vi "Find Supporting.vi"(11 "Bricks in":T1(array[cluster])) -> (3 "Bricks out":T1(array[cluster]))   [LabVIEW 2023, in "d22.lvlib"]
uses:
  d22.lvlib
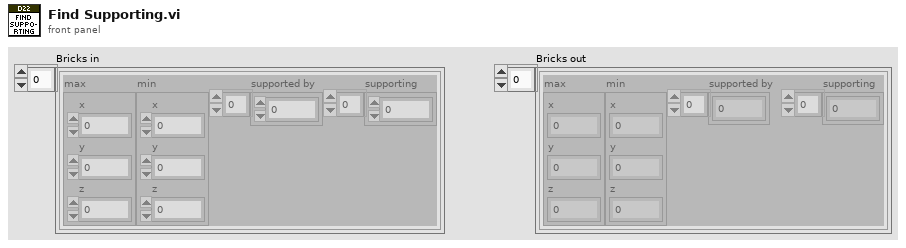
[diagram p1: front panel]
types:
  T1 = cluster{"max":cluster{"x":i32, "y":i32, "z":i32}, "min":cluster{"x":i32, "y":i32, "z":i32}, "supported by":i32[], "supporting":i32[]}[]
  T2 = cluster{"max":cluster{"x":i32, "y":i32, "z":i32}, "min":cluster{"x":i32, "y":i32, "z":i32}, "supported by":i32[], "supporting":i32[]}
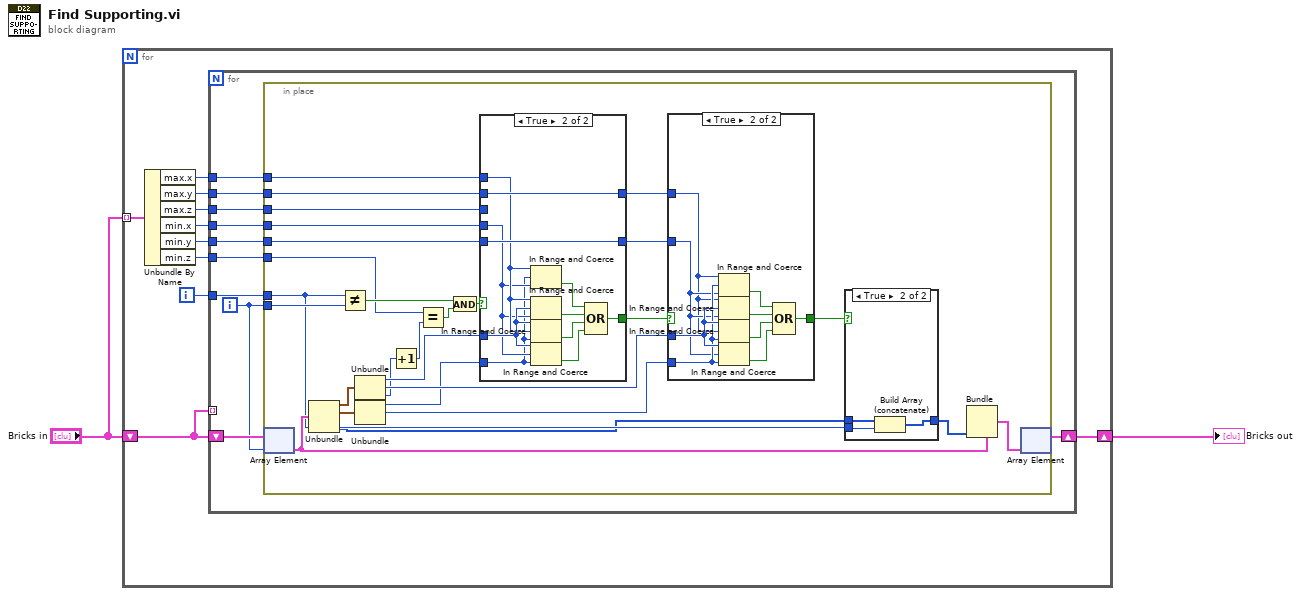
[diagram p0: block diagram]
diagram:
  n1 = for {
    shift-right: [w11] -> w2
    shift-left: "Bricks in" -> [w3]
    tunnel: "Bricks in" -> [w10] mode=indexing
    i -> [w12]
    n2 = Unbundle By Name(w10) -> ("max.x"=w8:i32, "max.y"=w9:i32, "max.z"=w7:i32, "min.x"=w6:i32, "min.y"=w5:i32, "min.z"=w4:i32)
    n3 = for {
      tunnel: w9 -> [w21]
      tunnel: w8 -> [w22]
      tunnel: w7 -> [w20]
      tunnel: w6 -> [w19]
      tunnel: w5 -> [w18]
      tunnel: w4 -> [w17]
      tunnel: w12 -> [w16]
      shift-right: [w13] -> w11
      shift-left: w3 -> [w15]
      tunnel: w3 -> [_] mode=indexing
      i -> [w14]
      n4 = in-place {
        in-place-border: w22 -> [w47]
        in-place-border: w21 -> [w46]
        in-place-border: w20 -> [w27]
        in-place-border: w19 -> [w45]
        in-place-border: w18 -> [w44]
        in-place-border: w17 -> [w25]
        in-place-border: w16 -> [w29]
        in-place-border: w14 -> [w32]
        n5 = in-place-array #1(w15, w14) -> (w31:T2)
        n6 = Unbundle(w31) -> ("max"=w49:cluster{"x":i32, "y":i32, "z":i32}, "min"=w48:cluster{"x":i32, "y":i32, "z":i32}, "supporting"=w24:i32[])  [unwired: 1 out]
        n7 = Not Equal?(x=w29, y=w32) -> (x != y?=w38:bool)
        n8 = Unbundle(w49) -> ("x"=w37:i32, "y"=w36:i32, "z"=w26:i32)
        n9 = Unbundle(w48) -> ("x"=w34:i32, "y"=w35:i32)  [unwired: 1 out]
        n10 = Increment(x=w26) -> (x+1=w28:i32)
        n11 = Equal?(x=w25, y=w28) -> (x = y?=w43:bool)
        n12 = And(x=w38, y=w43) -> (x .and. y?=w39:bool)
        n13 = case shown="True" w39 {
          tunnel: w47 -> [_ w72]
          tunnel: w46 -> [w64 w75]
          tunnel: w27 -> [_ _]
          tunnel: w45 -> [_ w71]
          tunnel: w44 -> [w63 w74]
          tunnel: [_ w65] -> w40
          tunnel: [w64 w75] -> w41
          tunnel: [w63 w74] -> w42
          tunnel: w37 -> [_ w73]
          tunnel: w34 -> [_ w70]
          frame False {
          }
          frame True {
            n14 = In Range and Coerce(upper limit=w72, x=w70, lower limit=w71) -> (In Range?=w66:bool)  [unwired: 1 out]
            n15 = In Range and Coerce(upper limit=w72, x=w73, lower limit=w71) -> (In Range?=w68:bool)  [unwired: 1 out]
            n16 = In Range and Coerce(upper limit=w73, x=w72, lower limit=w70) -> (In Range?=w69:bool)  [unwired: 1 out]
            n17 = In Range and Coerce(upper limit=w73, x=w71, lower limit=w70) -> (In Range?=w67:bool)  [unwired: 1 out]
            n18 = Compound Arithmetic op=OR(w66, w68, w69, w67) -> (w65:bool)
          }
        }
        n19 = case shown="True" w40 {
          tunnel: w41 -> [_ w54]
          tunnel: w42 -> [_ w55]
          tunnel: [_ w56] -> w33
          tunnel: w36 -> [_ w62]
          tunnel: w35 -> [_ w61]
          frame False {
          }
          frame True {
            n20 = In Range and Coerce(upper limit=w54, x=w61, lower limit=w55) -> (In Range?=w57:bool)  [unwired: 1 out]
            n21 = In Range and Coerce(upper limit=w54, x=w62, lower limit=w55) -> (In Range?=w59:bool)  [unwired: 1 out]
            n22 = In Range and Coerce(upper limit=w62, x=w54, lower limit=w61) -> (In Range?=w60:bool)  [unwired: 1 out]
            n23 = In Range and Coerce(upper limit=w62, x=w55, lower limit=w61) -> (In Range?=w58:bool)  [unwired: 1 out]
            n24 = Compound Arithmetic op=OR(w57, w59, w60, w58) -> (w56:bool)
          }
        }
        n25 = case shown="True" w33 {
          tunnel: w24 -> [w50 w53]
          tunnel: [w50 w52] -> w23
          tunnel: w29 -> [_ w51]
          frame False {
          }
          frame True {
            n26 = Build Array (concatenate)(w53, w51) -> (w52:i32[])
          }
        }
        n27 = Bundle(cluster=w31, "supporting"=w23) -> (w30:T2)  [unwired: 3 in]
        n28 = in-place-array #1(w30) -> (w13:T1)  [unwired: 1 out]
      }
    }
  }
  "Bricks out" <- w2
